vi "Get extended drive status.vi"(4 "Drive address":T4=1 items=["0", "1", "2", "3", "4", "5", "6", "7", "8", "9", "10", "11", "12", "13", "14", "15", "16", "17", "18", "19", "20", "21", "22", "23", "24", "25", "26", "27", "28", "29", "30", "31", "32", "33", "34", "35", "36", "37", "38", "39", "40", "41", "42", "43", "44", "45", "46", "47", "48", "49", "50", "51", "52", "53", "54", "55", "56", "57", "58", "59", "60", "61", "62", "63"], 5 "COM port":refnum<visa-resource-name>) -> (0 "Extended drive status":T3, 1 "Modbus error cluster":T1={"Checksum ok"=FALSE, "Modbus exception code"=1, "Response from correct drive"=FALSE, "Comms error"={"status"=FALSE, "code"=0, "source"=""}} {"Modbus exception code" items=["None"=0, "Invalid function request"=1, "Invalid Modbus register address"=2, "Invalid / unauthorised data value"=3, "Device failure"=4, "Request accepted, wait"=5, "Drive busy"=6, "Request rejected"=7, "Memory parity error"=8, "Gateway path unavailable"=10, "Device failed to respond"=11]}, 2 "No errors":bool)   [LabVIEW 2020]
doc: "Modbus RTU for Invertek drives. Paul Nathan 21-JUN-2022."
uses:
  ctls/Drive address.ctl
  ctls/Extended drive status bits.ctl
  ctls/Register.ctl
  ctls/Exception codes.ctl
  ctls/Modbus error cluster.ctl
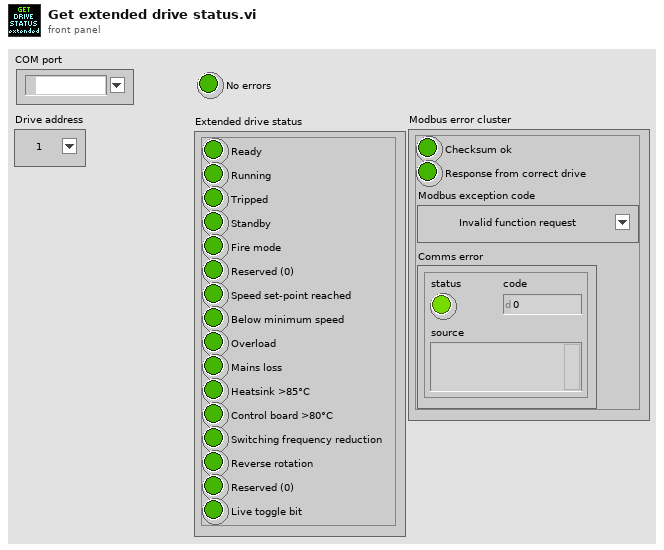
[diagram p1: front panel]
types:
  T1 = typedef "Modbus error cluster.ctl" = cluster{"Checksum ok":bool, "Modbus exception code":T2, "Response from correct drive":bool, "Comms error":errorcluster}
  T2 = typedef "Exception codes.ctl" = u8
  T3 = typedef "Extended drive status bits.ctl" = cluster{"Ready":bool, "Running":bool, "Tripped":bool, "Standby":bool, "Fire mode":bool, "Reserved (0)":bool, "Speed set-point reached":bool, "Below minimum speed":bool, "Overload":bool, "Mains loss":bool, "Heatsink >85°C":bool, "Control board >80°C":bool, "Switching frequency reduction":bool, "Reverse rotation":bool, "Reserved (0)":bool, "Live toggle bit":bool}
  T4 = typedef "Drive address.ctl" = u8
  T5 = typedef "Register.ctl" = u16
  T6 = cluster{"Boolean array[0]":bool, "Boolean array[1]":bool, "Boolean array[2]":bool, "Boolean array[3]":bool, "Boolean array[4]":bool, "Boolean array[5]":bool, "Boolean array[6]":bool, "Boolean array[7]":bool, "Boolean array[8]":bool, "Boolean array[9]":bool, "Boolean array[10]":bool, "Boolean array[11]":bool, "Boolean array[12]":bool, "Boolean array[13]":bool, "Boolean array[14]":bool, "Boolean array[15]":bool}
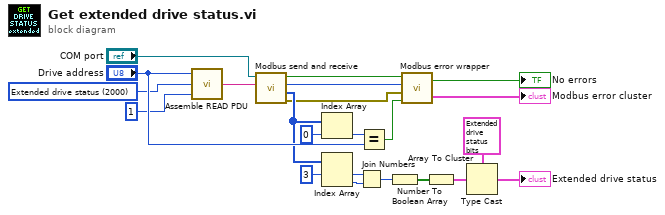
[diagram p0: block diagram]
diagram:
  w7 = T5 2000 items=["Control"=0, "RPM set-point"=4, "Drive status"=5, "Output RPM"=6, "Motor current"=7, "Motor torque"=8, "Motor power"=9, "DC bus voltage"=22, "Drive power stage temperature"=23, "kWh meter"=31, "MWh meter"=32, "Running time - hours"=33, "Running time - seconds"=34, "Internal drive temperature"=38, "Motor RMS voltage"=42, "Extended drive status"=2000] ("Register")
  n1 = call "Assemble READ PDU.vi"("No. of registers"=u16 1, "Register"=w7, "Drive address"="Drive address") -> ("Ser out string"=w22:string)
  n2 = call "Modbus send and receive.vi"("Modbus telegram"=w22, "COM port"="COM port") -> ("Comms error"=w2:errorcluster, "Device response"=w16:u8[], "Modbus exception code"=w1:T2, "Checksum ok"=w4:bool)  [unwired: 2 in]
  n3 = Index Array(array=w16, index=0) -> (element=w19:u8)
  n4 = Index Array(array=w16, index #1=3 ("index")) -> (element #1=w11:u8, element #2=w10:u8)  [unwired: 1 in]
  n5 = Join Numbers(hi=w11, lo=w10) -> ((hi.lo)=w9:u16)
  n6 = Equal?(x=w19, y="Drive address") -> (x = y?=w3:bool)
  n7 = Number To Boolean Array(number=w9) -> (Boolean array=w14:bool[])
  n8 = call "Modbus error wrapper.vi"("Response from correct drive"=w3, "Comms error"=w2, "Modbus exception code"=w1, "Checksum ok"=w4) -> ("Modbus error cluster"=→"Modbus error cluster":T1, "No errors"=→"No errors":bool)
  n9 = Array To Cluster(array=w14) -> (cluster=w13:T6)
  n10 = Type Cast(type=T3 {"Ready"=FALSE, "Running"=FALSE, "Tripped"=FALSE, "Standby"=FALSE, "Fire mode"=FALSE, "Reserved (0)"=FALSE, "Speed set-point reached"=FALSE, "Below minimum speed"=FALSE, "Overload"=FALSE, "Mains loss"=FALSE, "Heatsink >85°C"=FALSE, "Control board >80°C"=FALSE, "Switching frequency reduction"=FALSE, "Reverse rotation"=FALSE, "Reserved (0)"=FALSE, "Live toggle bit"=FALSE} ("Extended drive status"), x=w13) -> (*(type *) &x=→"Extended drive status":T3)
